vi "AMC Multiple Targets Example 2 (RT).vi"() -> ()   [LabVIEW 2014]
uses:
  vi.lib/NI/AMC/AMC.lvlib
panel:
  in  "UDP Port":u16=9000
  in  "Exit":bool
  out "Process":bool
  out "Status":string
  in  "State Variables":cluster{"CurrentFile":path}
  # "Target 2"
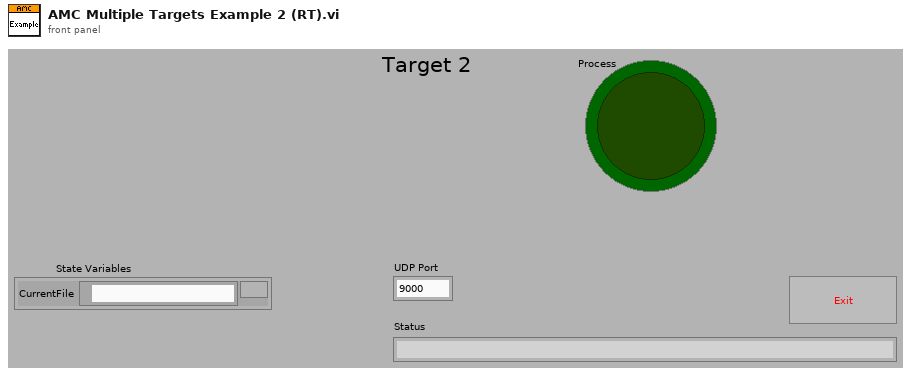
[diagram p1: front panel]
types:
  T1 = typedef "AMC.lvlib/Message Queue.ctl" = refnum<queue>
  T2 = typedef "AMC.lvlib/Message.ctl" = cluster{"name":string, "value":string, "attributes":T3, "receiver host":string, "receiver process":string, "source host":string, "source process":string, "priority message":bool, "acknowledge message":bool}
  T3 = typedef "Tools_KeyedArray.lvlib/KeyedArray.ctl" = cluster{"keys":string[], "values":string[]}
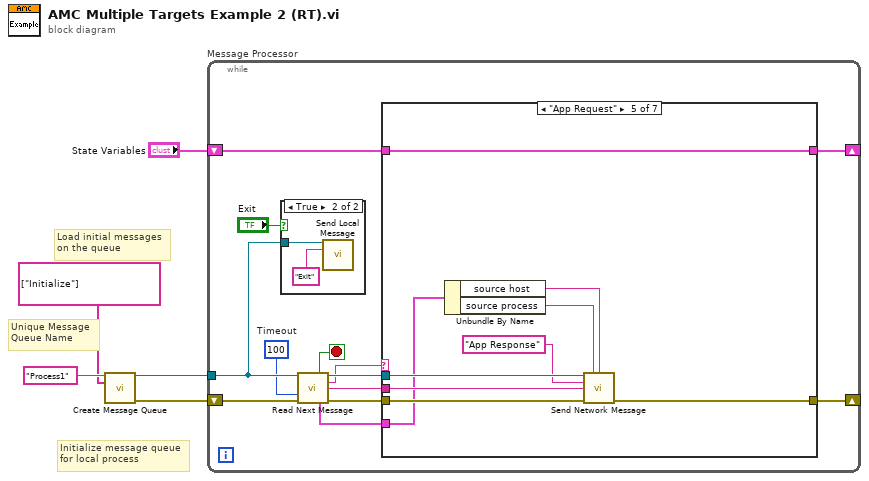
[diagram p0: block diagram]
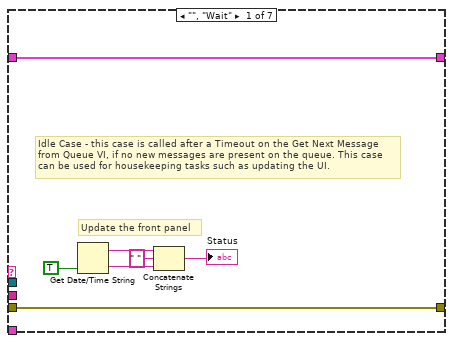
[diagram p3: hidden frame]
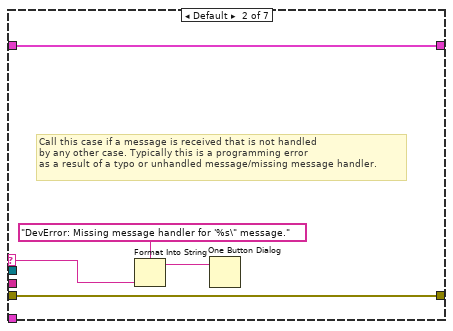
[diagram p4: hidden frame]
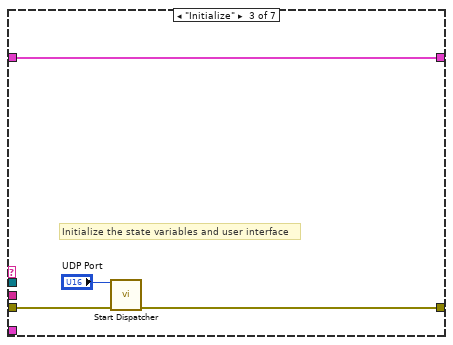
[diagram p5: hidden frame]
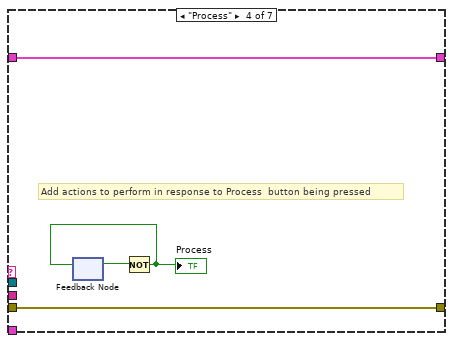
[diagram p6: hidden frame]
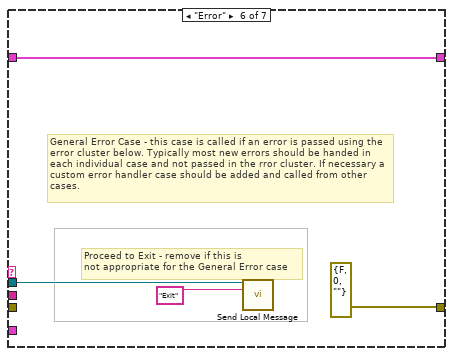
[diagram p7: hidden frame]
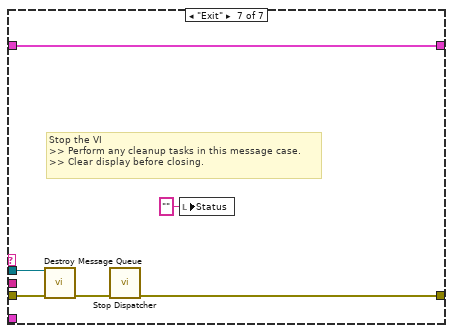
[diagram p8: hidden frame]
diagram:
  # "Initialize message queue\nfor local process"
  # "Unique Message\nQueue Name"
  # "Load initial messages\non the queue"
  n1 = call "Create Message Queue.vi"("message queue name"="Process1" ("Message queue name (unnamed)"), "initial message names"=string[] ["Initialize"]) -> ("message queue out"=w4:T1, "error out"=w2:errorcluster)  [unwired: 12 in]
  n2 = while "Message Processor" {
    shift-left: w2 -> [w13]
    shift-right: [w14] -> _
    tunnel: w4 -> [w9]
    shift-left: "State Variables" -> [w18]
    shift-right: [w17] -> _
    stop <- w11 stop-if-true
    w8 = 100  # Timeout
    n3 = case shown="True" "Exit" {
      tunnel: w9 -> [_ w19]
      frame False {
      }
      frame True {
        n4 = call "Send Local Message.vi"("message queue in"=w19, "message name"="Exit") -> ()  [unwired: 11 in, 3 out]
      }
    }
    n5 = call "Read Next Message.vi"("message queue in"=w9, "timeout (1 ms)"=w8, "error in"=w13) -> ("exit process?"=w11:bool, "message queue out"=w16:T1, "message name"=w12:string, "message value"=w7:string, "message"=w6:T2, "error out"=w15:errorcluster)  [unwired: 5 in, 2 out]
    n6 = case shown="\"App Request\"" w12 {
      selector: w12 -> [_ w30 _ _ _ _ _]
      tunnel: [w27 w32 w36 w39 w49 w53 w59] -> w17
      tunnel: w18 -> [w27 w32 w36 w39 w49 w53 w59]
      tunnel: w16 -> [_ _ _ _ w46 w51 w57]
      tunnel: w15 -> [w26 w31 w35 w40 w48 _ w56]
      tunnel: [w26 w31 w34 w40 w47 errorcluster {"status"=FALSE, "code"=0, "source"=""} ("error out") w54] -> w14
      tunnel: w7 -> [_ _ _ _ w44 _ _]
      tunnel: w6 -> [_ _ _ _ w43 _ _]
      frame "", "Wait" {
        # "Update the front panel"
        # "Idle Case - this case is called after a Timeout on the Get Next Message from Queue VI, if no new messages are present on the queue. This case can be used for housekeeping tasks such as updating the UI."
        n7 = Get Date/Time String(want seconds? (F)=TRUE) -> (date string=w25:string, time string=w24:string)  [unwired: 2 out]
        n8 = Concatenate Strings(w25, " " ("string"), w24) -> (→"Status":string)
      }
      frame Default {
        # "Call this case if a message is received that is not handled \nby any other case. Typically this is a programming error\nas a result of a typo or unhandled message/missing message handler."
        n9 = Format Into String(format string="DevError: Missing message handler for '%s\" message." ("message"), w30) -> (resulting string=w28:string)  [unwired: 2 in, 1 out]
        n10 = One Button Dialog(message=w28) -> ()  [unwired: 2 out]
      }
      frame "Initialize" {
        # "Initialize the state variables and user interface"
        n11 = call "Start Dispatcher.vi"("UDP port (0)"="UDP Port", "error in"=w35) -> ("error out"=w34:errorcluster)  [unwired: 11 in, 2 out]
      }
      frame "Process" {
        # "Add actions to perform in response to Process  button being pressed"
        n12 = feedback #1() -> (w38:bool)  [unwired: 1 out]
        n13 = Not(x=w38) -> (.not. x?=w37:bool)
        "Process" <- w37
        n14 = feedback-in #1(w37) -> ()
      }
      frame "App Request" {
        n15 = Unbundle By Name(w43) -> ("source host"=w42:string, "source process"=w41:string)
        n16 = call "Send Network Message.vi"("message queue in"=w46, "receiver process"=w41, "receiver host"=w42, "message name"="App Response", "message value"=w44, "error in"=w48) -> ("error out"=w47:errorcluster)  [unwired: 7 in, 2 out]
      }
      frame "Error" {
        # "Proceed to Exit - remove if this is\nnot appropriate for the General Error case"
        # "General Error Case - this case is called if an error is passed using the error cluster below. Typically most new errors should be handed in each individual case and not passed in the rror cluster. If necessary a custom error handler case should be added and called from other cases."
        n17 = call "Send Local Message.vi"("message queue in"=w51, "message name"="Exit") -> ()  [unwired: 11 in, 3 out]
      }
      frame "Exit" {
        # "Stop the VI\n>> Perform any cleanup tasks in this message case.\n>> Clear display before closing."
        n18 = call "Destroy Message Queue.vi"("message queue in"=w57, "error in"=w56) -> ("error out"=w55:errorcluster)  [unwired: 11 in, 2 out]
        n19 = call "Stop Dispatcher.vi"("error in"=w55) -> ("error out"=w54:errorcluster)  [unwired: 14 in]
        n20 = local write "Status"("" ("Status")) -> ()
      }
    }
  }
